vi "BooleanToBinary.vi"(11 "data":bool[](array[boolean])) -> (3 "BinaryOut":string)   [LabVIEW 2011]
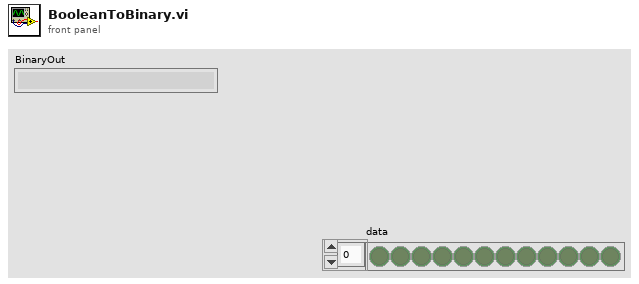
[diagram p1: front panel]
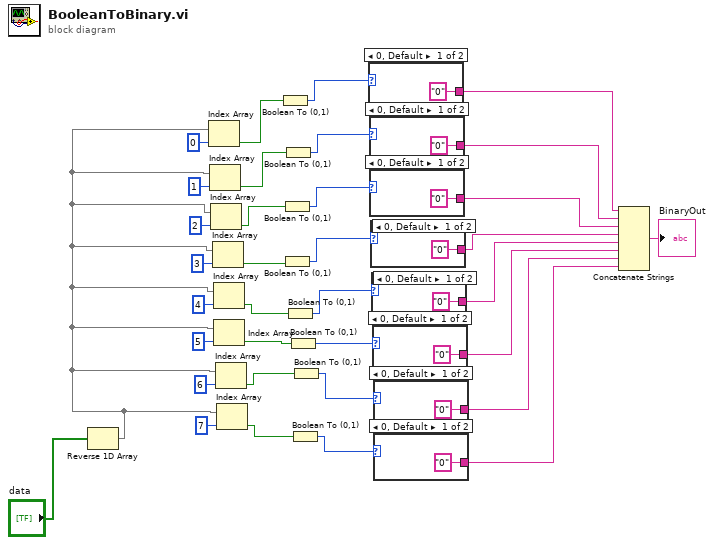
[diagram p0: block diagram]
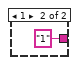
[diagram p2: hidden frame]
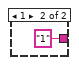
[diagram p3: hidden frame]
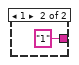
[diagram p4: hidden frame]
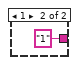
[diagram p5: hidden frame]
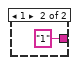
[diagram p6: hidden frame]
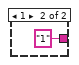
[diagram p7: hidden frame]
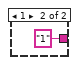
[diagram p8: hidden frame]
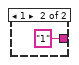
[diagram p9: hidden frame]
diagram:
  n1 = Reverse 1D Array(array="data") -> (reversed array=w2:bool[])
  n2 = Index Array(array=w2, index=0) -> (element=w27:bool)
  n3 = Index Array(array=w2, index=1) -> (element=w25:bool)
  n4 = Index Array(array=w2, index=2) -> (element=w24:bool)
  n5 = Index Array(array=w2, index=3) -> (element=w20:bool)
  n6 = Index Array(array=w2, index=4) -> (element=w19:bool)
  n7 = Index Array(array=w2, index=5) -> (element=w17:bool)
  n8 = Index Array(array=w2, index=6) -> (element=w15:bool)
  n9 = Index Array(array=w2, index=7) -> (element=w13:bool)
  n10 = Boolean To (0,1)(Boolean=w27) -> (0, 1=w26:i16)
  n11 = Boolean To (0,1)(Boolean=w24) -> (0, 1=w22:i16)
  n12 = Boolean To (0,1)(Boolean=w20) -> (0, 1=w21:i16)
  n13 = Boolean To (0,1)(Boolean=w25) -> (0, 1=w23:i16)
  n14 = Boolean To (0,1)(Boolean=w19) -> (0, 1=w18:i16)
  n15 = Boolean To (0,1)(Boolean=w17) -> (0, 1=w16:i16)
  n16 = Boolean To (0,1)(Boolean=w13) -> (0, 1=w12:i16)
  n17 = Boolean To (0,1)(Boolean=w15) -> (0, 1=w14:i16)
  n18 = case shown="0, Default" w26 {
    tunnel: ["0" ("decimal integer string") "1" ("decimal integer string")] -> w11
    frame 0, Default {
    }
    frame 1 {
    }
  }
  n19 = case shown="0, Default" w23 {
    tunnel: ["0" ("decimal integer string") "1" ("decimal integer string")] -> w10
    frame 0, Default {
    }
    frame 1 {
    }
  }
  n20 = case shown="0, Default" w22 {
    tunnel: ["0" ("decimal integer string") "1" ("decimal integer string")] -> w9
    frame 0, Default {
    }
    frame 1 {
    }
  }
  n21 = case shown="0, Default" w21 {
    tunnel: ["0" ("decimal integer string") "1" ("decimal integer string")] -> w8
    frame 0, Default {
    }
    frame 1 {
    }
  }
  n22 = case shown="0, Default" w18 {
    tunnel: ["0" ("decimal integer string") "1" ("decimal integer string")] -> w7
    frame 0, Default {
    }
    frame 1 {
    }
  }
  n23 = case shown="0, Default" w16 {
    tunnel: ["0" ("decimal integer string") "1" ("decimal integer string")] -> w6
    frame 0, Default {
    }
    frame 1 {
    }
  }
  n24 = case shown="0, Default" w14 {
    tunnel: ["0" ("decimal integer string") "1" ("decimal integer string")] -> w5
    frame 0, Default {
    }
    frame 1 {
    }
  }
  n25 = case shown="0, Default" w12 {
    tunnel: ["0" ("decimal integer string") "1" ("decimal integer string")] -> w4
    frame 0, Default {
    }
    frame 1 {
    }
  }
  n26 = Concatenate Strings(w11, w10, w9, w8, w7, w6, w5, w4) -> (→"BinaryOut":string)
